vi "tunable_lenses_with_delay.vi"(7 "Delay (milliseconds)":u16, 8 "Tuneable Lens 4":T1 max=40000 step=1, 9 "Tuneable Lens 3":T1 max=40000 step=1, 10 "Tuneable Lens 2":T2 max=40000 step=1 scale=0.0..40000.0, 11 "Tuneable Lens 1":T2 max=40000 step=1 scale=0.0..40000.0) -> ()   [LabVIEW 2013]
uses:
  Tunable_Lens_Slider_Control.ctl
  Tuneable_Lens_Numeric_Control.ctl
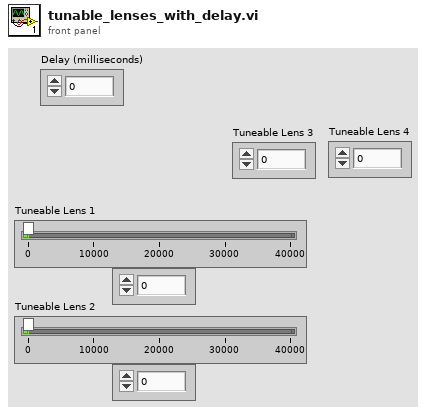
[diagram p1: front panel]
types:
  T1 = typedef "Tuneable_Lens_Numeric_Control.ctl" = u16
  T2 = typedef "Tunable_Lens_Slider_Control.ctl" = u16
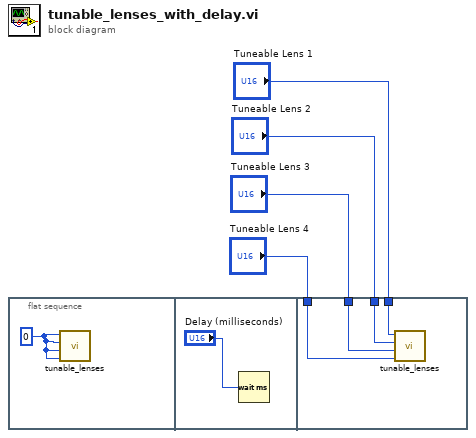
[diagram p0: block diagram]
diagram:
  n1 = flat-sequence {
    tunnel: "Tuneable Lens 1" -> [w10]
    tunnel: "Tuneable Lens 2" -> [w9]
    tunnel: "Tuneable Lens 3" -> [w8]
    tunnel: "Tuneable Lens 4" -> [w7]
    frame #0 {
      w5 = u16 0 ("DAC1")
      n2 = call "tunable_lenses.vi"("DAC4"=w5, "DAC3"=w5, "DAC2"=w5, "DAC1"=w5) -> ()  [unwired: 7 in, 1 out]
    }
    frame #1 {
      n3 = Wait (ms)(milliseconds to wait="Delay (milliseconds)") -> ()  [unwired: 1 out]
    }
    frame #2 {
      n4 = call "tunable_lenses.vi"("DAC4"=w7, "DAC3"=w8, "DAC2"=w9, "DAC1"=w10) -> ()  [unwired: 7 in, 1 out]
    }
  }
